vi "create_folder.vi"(9 "Input \nparameters":T2={"Frame rate (ms)"=2000, "Worm strain"="N2", "# Images"=0, "State"=enum."Image acquisition", "Time elapsed"=0.0, "Max_num_runs"=100000, "#TTL"=0, "Time of start TTL"=100000, "ImSub Value"=0, "Time of last TTL"=0, "Number of Columns"=2, "Number of Rows"=2, "# AdjacentTTL"=0, "Sleep deprivation status"="", "Sleep Detection"=FALSE, "# Sleep detections"=0, "Time of first sleep detection"=0, "Time max # adjacent TTL"=0, "Image t-1"=[], "Image t"=[]} {"Number of Rows" items=["1"=1, "2"=2, "3"=3, "4"=4]; "Number of Columns" items=["1"=1, "2"=2, "3"=3, "4"=4]}) -> ()   [LabVIEW 2011]
uses:
  state.ctl
  Action Items.ctl
  Action-Init-Update-Get.ctl
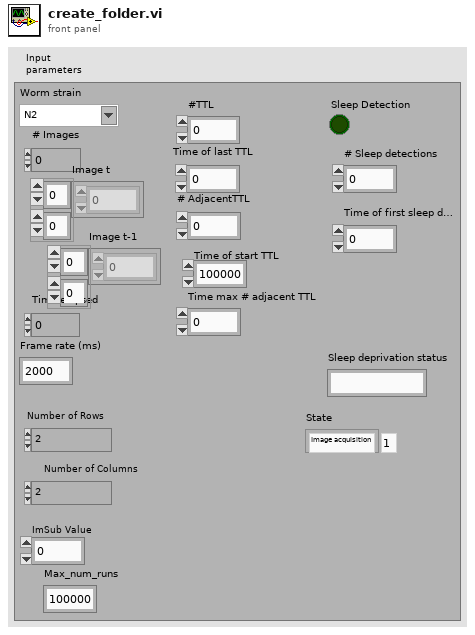
[diagram p1: front panel]
types:
  T1 = typedef "state.ctl" = enum16{"Initialize measurement", "Image acquisition", "Image processing", "Sleep detection", "Control TTL protocol ", "Sleep deprivation", "Update image & exit condition", "Wait "}
  T2 = cluster{"Frame rate (ms)":u32, "Worm strain":string, "# Images":i32, "State":T1, "Time elapsed":dbl, "Max_num_runs":i32, "#TTL":i32, "Time of start TTL":i32, "ImSub Value":i32, "Time of last TTL":i32, "Number of Columns":u32, "Number of Rows":u32, "# AdjacentTTL":i32, "Sleep deprivation status":string, "Sleep Detection":bool, "# Sleep detections":i32, "Time of first sleep detection":i32, "Time max # adjacent TTL":i32, "Image t-1":i32[][], "Image t":i32[][]}
  T3 = typedef "Action Items.ctl" = enum16{"Initialize", "Get"}
  T4 = typedef "Action-Init-Update-Get.ctl" = enum16{"Initialize", "Update", "Get"}
  T5 = cluster{"Path":string, "Filestem":string, "Filestem incl time t":string, "Date":string}
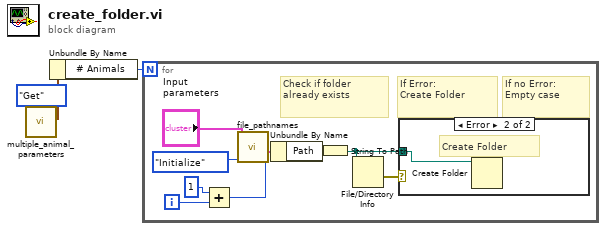
[diagram p0: block diagram]
diagram:
  n1 = call "multiple_animal_parameters.vi"("Action"=Action_Items."Get") -> ("Animal\nparameters"=w2:cluster{"# Animals":i32, "Index SD animal":i32})  [unwired: 10 in]
  n2 = Unbundle By Name(w2) -> ("# Animals"=w1:i32)
  n3 = for {
    N: w1 -> [_]
    i -> [w8]
    # "If Error:\nCreate Folder"
    # "If no Error:\nEmpty case"
    # "Check if folder\nalready exists"
    n4 = Add(x=1, y=w8) -> (x+y=w6:i32)
    n5 = call "file_pathnames.vi"("Animal x"=w6, "Action"=Action-Init-Update-Get."Initialize", "Input \nparameters"="Input \nparameters") -> ("File-path\n-names"=w9:T5)  [unwired: 8 in]
    n6 = Unbundle By Name(w9) -> ("Path"=w10:string)
    n7 = String To Path(string=w10) -> (path=w11:path)
    n8 = File/Directory Info(path=w11) -> (error out=w12:errorcluster)  [unwired: 1 in, 6 out]
    n9 = case shown="Error" w12 {
      tunnel: w11 -> [_ w13]
      frame No Error {
      }
      frame Error {
        # "Create Folder"
        n10 = Create Folder(path (use dialog)=w13) -> ()  [unwired: 2 in, 3 out]
      }
    }
  }
